vi "8164B Attenuators Enable.vi"(7 "Slots":string[](array[string]), 8 "error in":errorcluster, 10 "Enable":bool, 11 "KeySight 8164B control in":T1) -> (0 "error out":errorcluster, 3 "KeySight 8164B control out":T1)   [LabVIEW 2018, in "KeySight 8164B LAN InstrLib.lvlib"]
uses:
  KeySight 8164B LAN InstrLib.lvlib
  typedefs/KeySight 8164B control.ctl
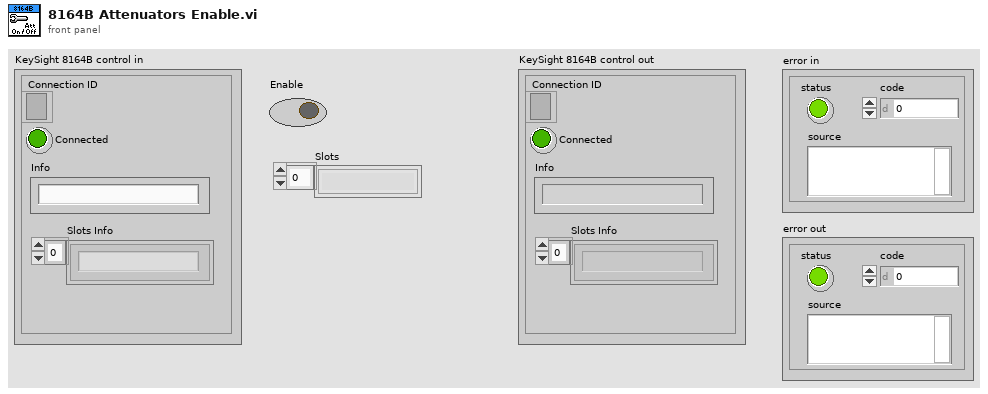
[diagram p1: front panel]
types:
  T1 = typedef "KeySight 8164B LAN InstrLib.lvlib/KeySight 8164B control.ctl" = cluster{"Connection ID":refnum<k5>, "Connected":bool, "Info":string, "Slots Info":string[]}
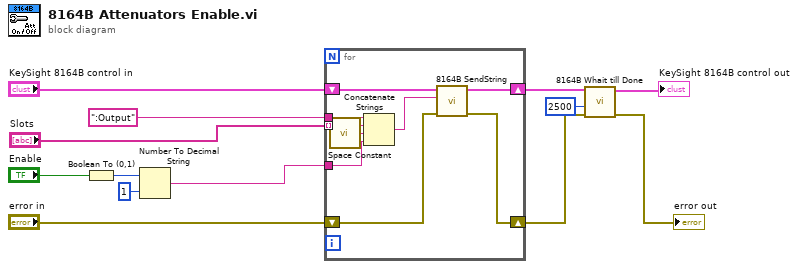
[diagram p0: block diagram]
diagram:
  n1 = Boolean To (0,1)(Boolean="Enable") -> (0, 1=w10:i16)
  n2 = Number To Decimal String(number=w10, width (-)=i16 1) -> (decimal integer string=w8:string)
  n3 = for {
    shift-right: [w21] -> w7
    shift-left: "KeySight 8164B control in" -> [w22]
    shift-right: [w19] -> w5
    shift-left: "error in" -> [w20]
    tunnel: w8 -> [w16]
    tunnel: "Slots" -> [w18] mode=indexing
    tunnel: ":Output" -> [w14]
    n4 = call <vilib>:"Space Constant.vi"() -> ("String"=w17:string)
    n5 = Concatenate Strings(w14, w18, w17, w16) -> (w15:string)
    n6 = call "8164B SendString.vi"("error in"=w20, "CMD"=w15, "KeySight 8164B control in"=w22) -> ("error out"=w19:errorcluster, "KeySight 8164B control out"=w21:T1)  [unwired: 7 in]
  }
  n7 = call "8164B Whait till Done.vi"("error in"=w5, "timeout ms"=2500, "KeySight 8164B control in"=w7) -> ("error out"=→"error out":errorcluster, "KeySight 8164B control out"=→"KeySight 8164B control out":T1)  [unwired: 7 in]
